vi "ToString.vi"(8 "error in (no error)":errorcluster, 11 "Test In":refnum<class "Test.lvclass">) -> (0 "error out":errorcluster, 2 "String":string, 3 "Test Out":refnum<class "Test.lvclass">)   [LabVIEW 2019, in "Test.lvclass"]
doc: "Returns the string representation for this object."
uses:
  Test.lvclass
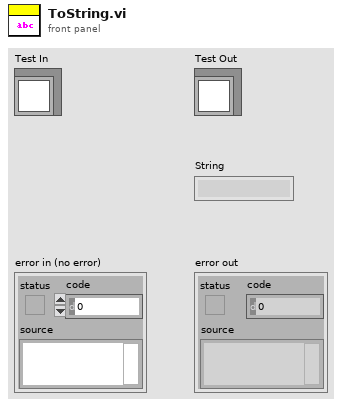
[diagram p1: front panel]
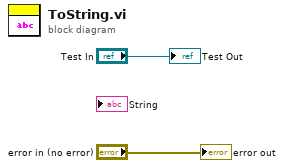
[diagram p0: block diagram]
diagram:
  "error out" <- "error in (no error)"
  "Test Out" <- "Test In"
